vi "模板读取.vi"(1 "Path":path) -> (0 "模板特征参数":dbl[][](array[numeric]))   [LabVIEW 2013]
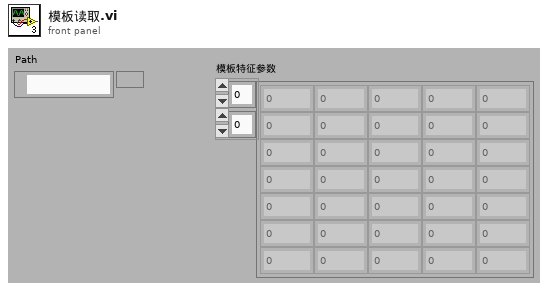
[diagram p1: front panel]
types:
  T1 = enum16{"open", "replace", "create", "open or create", "replace or create", "replace or create with confirmation"}
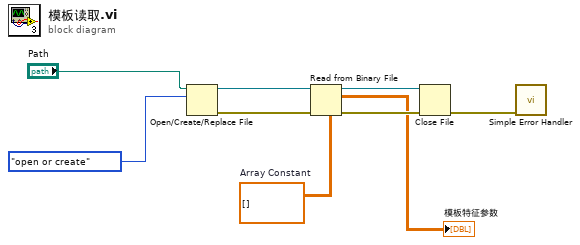
[diagram p0: block diagram]
diagram:
  w2 = dbl[][] []  # Array Constant
  n1 = Open/Create/Replace File(file path (use dialog)="Path", operation (0:open)=T1."open or create") -> (refnum out=w6:refnum<file>, error out=w7:errorcluster)  [unwired: 4 in, 1 out]
  n2 = Read from Binary File(5:w2, 8:w7, 11:w6) -> (0:w9:errorcluster, 2:→"模板特征参数":dbl[][], 3:w4:refnum<file>)  [unwired: 3 in, 1 out]
  n3 = Close File(refnum=w4, error in=w9) -> (error out=w8:errorcluster)  [unwired: 1 out]
  n4 = call <vilib>:"Simple Error Handler.vi"("error in (no error)"=w8) -> ()  [unwired: 4 in, 5 out]
